vi "FRCts20_Backend_Test_Event.vi"() -> ()   [LabVIEW 2014, in "FRCts20_Backend_TestCode.lvlib"]
uses:
  FRCts20_Backend_TestCode.lvlib
  FRCts20_Backend_API/FRCts20_Backend_API_Command_App.ctl
  FRCts20_Backend_API/FRCts20_Backend_API_EventRoot.ctl
  FRCts20_Backend_API/FRCts20_Backend_API_Event.ctl
  FRCts20_Backend_API/FRCts20_Backend_API_SW.ctl
  FRCts20_Backend_API/FRCts20_Backend_API_Application.vi
  FRCts20_Backend_API/FRCts20_Backend_API.lvlib
  FRCts20_Backend_Engine.lvlib
panel:
  out "Get Root Pass/Fail":bool
  out "Get Root":u32
  out "Get Pass/Fail":bool
  out "error out":errorcluster
  out "Del Pass/Fail":bool
  out "GetDel":u32
  out "Del":u32
  out "GetPut":u32
  out "Put":u32
  out "Put Pass/Fail":bool
  out "Post Pass/Fail":bool
  out "GetRootPost":u32
  out "post":u32
  out "Get":u32
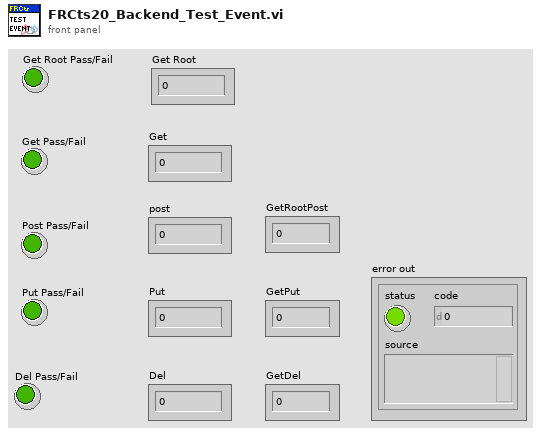
[diagram p1: front panel]
types:
  T1 = typedef "FRCts20_Backend_API.lvlib/FRCts20_Backend_API_Event.ctl" = cluster{"Event Index":u32, "Name":string, "Start Time":timestamp, "End Time":timestamp, "Teams":cluster{"Team Index":u32, "Team Number":u32, "Requests":cluster{"Request Number":u32, "Description":string}[], "Has Open Issue":bool}[], "SWType":T2, "APIReturn":string}
  T2 = typedef "FRCts20_Backend_API.lvlib/FRCts20_Backend_API_SW.ctl" = string
  T3 = typedef "FRCts20_Backend_API.lvlib/FRCts20_Backend_API_EventRoot.ctl" = cluster{"Event":cluster{"Event Index":u32, "EventID":u32, "EventSubtype":string, "EventSubtypeID":u32, "DistrictCode":string, "DistrictID":u32, "Event Name":string, "Venue":string, "City":string, "StateProvince":string, "Country":string, "Start Time":timestamp, "End Time":timestamp, "Year":u32, "NumberOfTeams":u32, "URLTeamlist":string, "EventCode":string, "OpenIssues":u8, "IsLive":bool}[], "APIReturn":string}
  T4 = typedef "FRCts20_Backend_API.lvlib/FRCts20_Backend_API_Command_App.ctl" = string
  T5 = cluster{"Event Index":u32, "EventID":u32, "EventSubtype":string, "EventSubtypeID":u32, "DistrictCode":string, "DistrictID":u32, "Event Name":string, "Venue":string, "City":string, "StateProvince":string, "Country":string, "Start Time":timestamp, "End Time":timestamp, "Year":u32, "NumberOfTeams":u32, "URLTeamlist":string, "EventCode":string, "OpenIssues":u8, "IsLive":bool}[]
  T6 = cluster{"Event Index":u32, "EventID":u32, "EventSubtype":string, "EventSubtypeID":u32, "DistrictCode":string, "DistrictID":u32, "Event Name":string, "Venue":string, "City":string, "StateProvince":string, "Country":string, "Start Time":timestamp, "End Time":timestamp, "Year":u32, "NumberOfTeams":u32, "URLTeamlist":string, "EventCode":string, "OpenIssues":u8, "IsLive":bool}
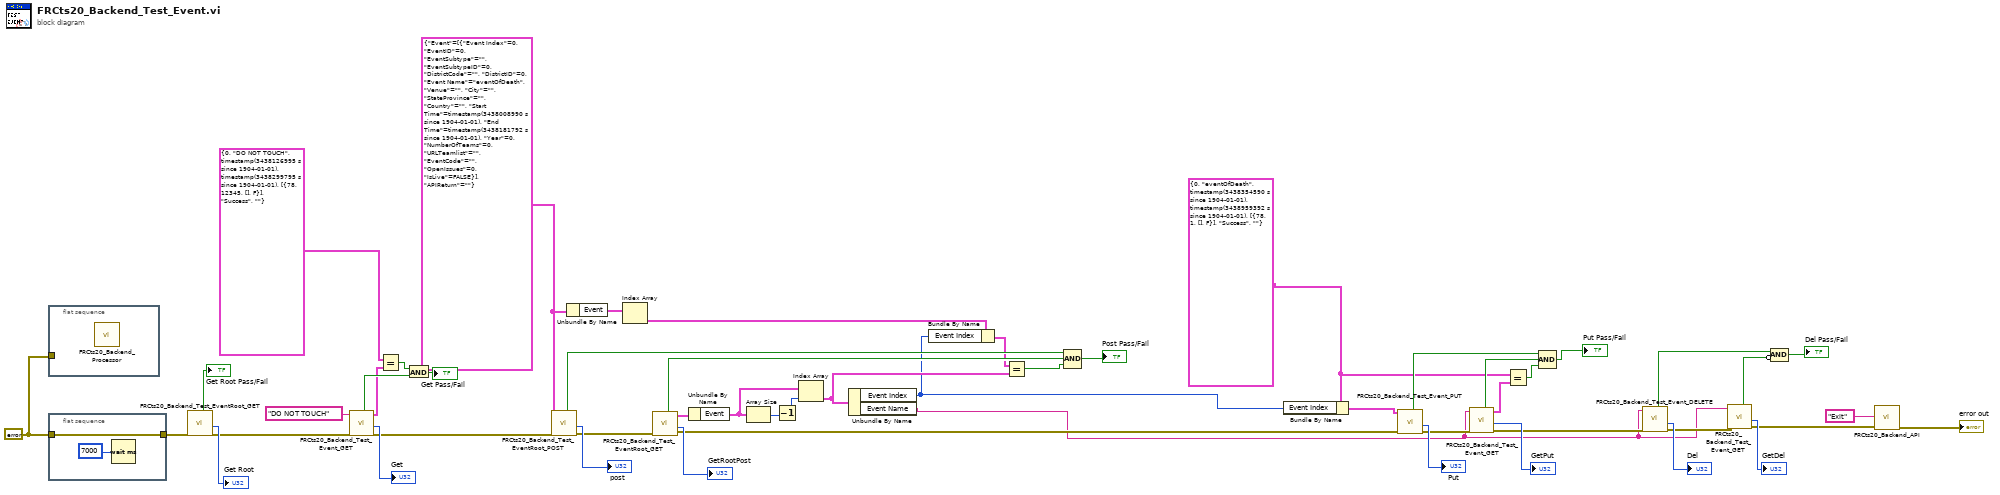
[diagram p0: block diagram]
diagram:
  w2 = T1 {"Event Index"=0, "Name"="eventOfDeath", "Start Time"=timestamp(3438354590 s since 1904-01-01), "End Time"=timestamp(3438959392 s since 1904-01-01), "Teams"=[{"Team Index"=78, "Team Number"=1, "Requests"=[], "Has Open Issue"=FALSE}], "SWType"="Success", "APIReturn"=""} ("Event Out")
  w5 = T3 {"Event"=[{"Event Index"=0, "EventID"=0, "EventSubtype"="", "EventSubtypeID"=0, "DistrictCode"="", "DistrictID"=0, "Event Name"="eventOfDeath", "Venue"="", "City"="", "StateProvince"="", "Country"="", "Start Time"=timestamp(3438008990 s since 1904-01-01), "End Time"=timestamp(3438181792 s since 1904-01-01), "Year"=0, "NumberOfTeams"=0, "URLTeamlist"="", "EventCode"="", "OpenIssues"=0, "IsLive"=FALSE}], "APIReturn"=""} ("EventRoot In")
  w51 = errorcluster {"status"=FALSE, "code"=0, "source"=""} ("error constant")
  n1 = flat-sequence {
    tunnel: w51 -> [_]
    frame #0 {
      n2 = call "FRCts20_Backend_Processor.vi"() -> ()  [unwired: 12 in]
    }
  }
  n3 = flat-sequence {
    tunnel: w51 -> [w53]
    tunnel: [w53] -> w49
    frame #0 {
      n4 = Wait (ms)(milliseconds to wait=u32 7000) -> ()  [unwired: 1 out]
    }
  }
  n5 = call "FRCts20_Backend_Test_EventRoot_GET.vi"("error in (no error)"=w49) -> ("error out"=w46:errorcluster, "Time (ms)"=→"Get Root":u32, "Success"=→"Get Root Pass/Fail":bool)  [unwired: 6 in, 2 out]
  n6 = call "FRCts20_Backend_Test_Event_GET.vi"("error in (no error)"=w46, "Name"="DO NOT TOUCH") -> ("error out"=w44:errorcluster, "Time (ms)"=→"Get":u32, "Event Out"=w8:T1, "Success"=w21:bool)  [unwired: 5 in, 1 out]
  n7 = Equal?(x=T1 {"Event Index"=0, "Name"="DO NOT TOUCH", "Start Time"=timestamp(3438126995 s since 1904-01-01), "End Time"=timestamp(3438299795 s since 1904-01-01), "Teams"=[{"Team Index"=78, "Team Number"=12345, "Requests"=[], "Has Open Issue"=FALSE}], "SWType"="Success", "APIReturn"=""} ("Event Out"), y=w8) -> (x = y?=w20:bool)
  n8 = And(x=w20, y=w21) -> (x .and. y?=→"Get Pass/Fail":bool)
  n9 = call "FRCts20_Backend_Test_EventRoot_POST.vi"("error in (no error)"=w44, "EventRoot In"=w5) -> ("error out"=w42:errorcluster, "Time (ms)"=→"post":u32, "Success"=w31:bool)  [unwired: 5 in, 2 out]
  n10 = Unbundle By Name(w5) -> ("Event"=w15:T5)
  n11 = Index Array(array=w15) -> (element=w13:T6)  [unwired: 1 in]
  n12 = call "FRCts20_Backend_Test_EventRoot_GET.vi"("error in (no error)"=w42) -> ("error out"=w40:errorcluster, "Time (ms)"=→"GetRootPost":u32, "Events"=w19:T3, "Success"=w30:bool)  [unwired: 6 in, 1 out]
  n13 = Unbundle By Name(w19) -> ("Event"=w16:T5)
  n14 = Array Size(array=w16) -> (size(s)=w18:i32)
  n15 = Decrement(x=w18) -> (x-1=w17:i32)
  n16 = Index Array(array=w16, index=w17) -> (element=w14:T6)
  n17 = Unbundle By Name(w14) -> ("Event Index"=w6:u32, "Event Name"=w1:string)
  n18 = Bundle By Name(cluster=w13, "Event Index"=w6) -> (w12:T6)
  n19 = Equal?(x=w12, y=w14) -> (x = y?=w29:bool)
  n20 = Compound Arithmetic op=AND(w31, w30, w29) -> (→"Post Pass/Fail":bool)
  n21 = Bundle By Name(cluster=w2, "Event Index"=w6) -> (w7:T1)
  n22 = call "FRCts20_Backend_Test_Event_PUT.vi"("error in (no error)"=w40, "Event Out"=w7) -> ("error out"=w38:errorcluster, "Time (ms)"=→"Put":u32, "Success"=w26:bool)  [unwired: 5 in, 2 out]
  n23 = call "FRCts20_Backend_Test_Event_GET.vi"("error in (no error)"=w38, "Name"=w1) -> ("error out"=w36:errorcluster, "Time (ms)"=→"GetPut":u32, "Event Out"=w23:T1, "Success"=w25:bool)  [unwired: 5 in, 1 out]
  n24 = Equal?(x=w2, y=w23) -> (x = y?=w24:bool)
  n25 = Compound Arithmetic op=AND(w26, w25, w24) -> (→"Put Pass/Fail":bool)
  n26 = call "FRCts20_Backend_Test_Event_DELETE.vi"("error in (no error)"=w36, "Event Name"=w1) -> ("error out"=w34:errorcluster, "Time (ms)"=→"Del":u32, "Success"=w11:bool)  [unwired: 5 in, 2 out]
  n27 = call "FRCts20_Backend_Test_Event_GET.vi"("error in (no error)"=w34, "Name"=w1) -> ("error out"=w32:errorcluster, "Time (ms)"=→"GetDel":u32, "Success"=w10:bool)  [unwired: 5 in, 2 out]
  n28 = Compound Arithmetic op=AND(w11, invert w10) -> (→"Del Pass/Fail":bool)
  n29 = call-poly "FRCts20_Backend_API.vi"("error in (no error)"=w32, "Command"=T4 "Exit") -> ("error out"=→"error out":errorcluster)  [unwired: 7 in, 2 out]
